vi "Unregister and Close Sessions.vi"(8 "error in":errorcluster) -> (0 "error out":errorcluster)   [LabVIEW 2021, in "DmmMeasurementHAL.lvlib"]
uses:
  DmmMeasurementHAL.lvlib
  <vilib>/Plug-In SDKs/Clients/Session Management V1/Session Reservation/Session Reservation.lvclass/Session Reservation.ctl
  <vilib>/Plug-In SDKs/Clients/Session Management V1/Session Reservation/Initialize and Close Session Behavior.ctl
  <vilib>/Plug-In SDKs/Clients/Session Management V1/Session Reservation/Merge Invalid DVR Error.vi
  <vilib>/Plug-In SDKs/Clients/Session Management V1/Session Reservation/Is DVR Valid.vi
  <vilib>/Plug-In SDKs/Measurements/Helpers/Error Strings Global Internal.vi
  <vilib>/Utility/error.llb/Error Cluster From Error Code.vi
  HAL/Instruments/DMM_Base/DMM_Base.lvclass
  HAL/Reusables/Get Pin Information.lvlib
  <vilib>/Plug-In SDKs/Clients/Session Management V1/Session Reservation/Session Reservation.lvclass
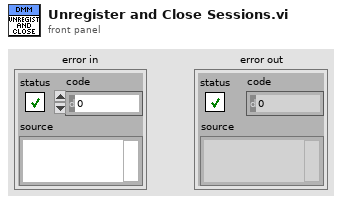
[diagram p1: front panel]
types:
  T1 = typedef "ni.measurementlink.sessionmanagement.v1.api.lvlib/ni_measurementlink_sessionmanagement_v1_SessionInformation.ctl" = cluster{"session":T2, "resource_name":string, "channel_list":string, "instrument_type_id":string, "session_exists":bool, "channel_mappings":T3[]}
  T2 = typedef "ni.measurementlink.sessionmanagement.v1.api.lvlib/nidevice_grpc_Session.ctl" = cluster{"name":string}
  T3 = typedef "ni.measurementlink.sessionmanagement.v1.api.lvlib/ni_measurementlink_sessionmanagement_v1_ChannelMapping.ctl" = cluster{"pin_or_relay_name":string, "site":i32, "channel":string, "multiplexer_resource_name":string, "multiplexer_route":string}
  T4 = typedef "NI Session Management V1 Client.lvlib/Session Reservation.lvclass/Initialize and Close Session Behavior.ctl" = enum16{"Auto", "Initialize and Close", "Attach and Detach", "Initialize and Detach", "Attach and Close"}
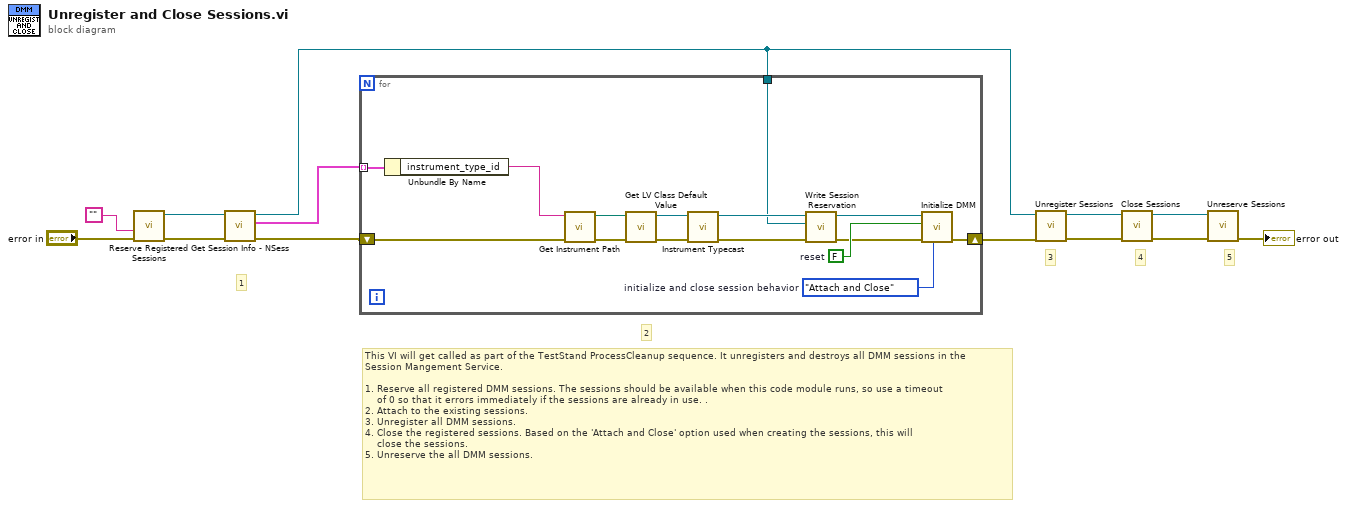
[diagram p0: block diagram]
diagram:
  # "5"
  # "4"
  # "3"
  # "2"
  # "1"
  # "This VI will get called as part of the TestStand ProcessCleanup sequence. It unregisters and destroys all DMM sessions in the\nSession Mangement Service.\n\n1. Reserve all registered DMM sessions. The sessions should be available when this code module runs, so use a timeout\n    of 0 so that it errors immediately if the sessions are already in use. .\n2. Attach to the existing sessions.\n3. Unregister all DMM sessions.\n4. Close the registered sessions. Based on the 'Attach and Close' option used when creating the sessions, this will\n    close the sessions.\n5. Unreserve the all DMM sessions."
  n1 = call <vilib>:"Reserve Registered Sessions.vi"("error in"="error in", "instrument type id"="") -> ("error out"=w10:errorcluster, "session reservation out"=w11:refnum<class "Session Reservation.lvclass">)  [unwired: 8 in]
  n2 = call <vilib>:"Get Session Info - NSess .vi"("error in"=w10, "session reservation in"=w11) -> ("error out"=w4:errorcluster, "sessions info"=w3:T1[], "session reservation out"=w2:refnum<class "Session Reservation.lvclass">)  [unwired: 7 in]
  n3 = for {
    shift-right: [w25] -> w1
    shift-left: w4 -> [w16]
    tunnel: w3 -> [w28] mode=indexing
    tunnel: w2 -> [w18]
    w23 = FALSE  # reset
    w24 = Initialize_and_Close_Session_Behavior."Attach and Close"  # initialize and close session behavior
    n4 = Unbundle By Name(w28) -> ("instrument_type_id"=w17:string)
    n5 = call "Get Instrument Path.vi"("error in"=w16, "instrument_type_id"=w17) -> ("error out"=w15:errorcluster, "Instrument Path"=w14:path)  [unwired: 8 in]
    n6 = call <vilib>:"Get LV Class Default Value.vi"("error in (no error)"=w15, "class path"=w14) -> ("error out"=w27:errorcluster, "object"=w26:refnum<class>)  [unwired: 8 in]
    n7 = call "Instrument Typecast.vi"("error in (no error)"=w27, "pin instrument"=w26) -> ("error out"=w22:errorcluster, "instrument object"=w19:refnum<class "DMM_Base.lvclass">)  [unwired: 8 in]
    n8 = call-dynamic "Write Session Reservation.vi"("error in (no error)"=w22, "Session Reservation"=w18, "DMM_Base in"=w19) -> ("error out"=w21:errorcluster, "DMM_Base out"=w20:refnum<class "DMM_Base.lvclass">)  [unwired: 7 in]
    n9 = call-dynamic "Initialize DMM.vi"("initialize and close session behavior"=w24, "error in (no error)"=w21, "reset"=w23, "DMM_Base in"=w20) -> ("error out"=w25:errorcluster)  [unwired: 6 in, 1 out]
  }
  n10 = call <vilib>:"Unregister Sessions.vi"("error in"=w1, "session reservation in"=w2) -> ("error out"=w6:errorcluster, "session reservation out"=w7:refnum<class "Session Reservation.lvclass">)  [unwired: 8 in]
  n11 = call <vilib>:"Close Sessions.vi"("error in"=w6, "session reservation in"=w7) -> ("error out"=w9:errorcluster, "session reservation out"=w8:refnum<class "Session Reservation.lvclass">)  [unwired: 8 in]
  n12 = call <vilib>:"Unreserve Sessions.vi"("error in"=w9, "session reservation in"=w8) -> ("error out"=→"error out":errorcluster)  [unwired: 9 in]
